vi "core_binary_split_DBL.vi"(9 "vector in":dbl[](array[numeric])) -> (0 "back":dbl[](array[numeric]), 1 "middle":dbl, 2 "front":dbl[](array[numeric]), 4 "odd length?":bool)   [LabVIEW 2015]
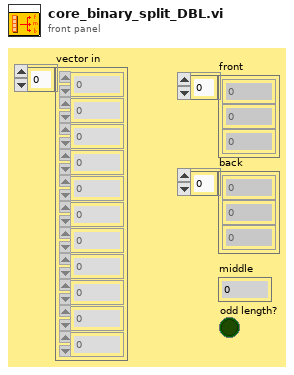
[diagram p1: front panel]
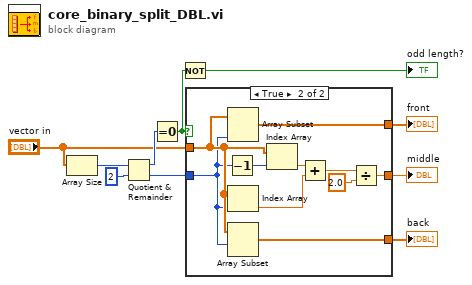
[diagram p0: block diagram]
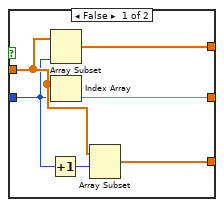
[diagram p2: hidden frame]
diagram:
  n1 = Array Size(array="vector in") -> (size(s)=w9:i32)
  n2 = Quotient & Remainder(x=w9, y=2) -> (x-y*floor(x/y)=w8:i32, floor(x/y)=w7:i32)
  n3 = Equal To 0?(x=w8) -> (x = 0?=w2:bool)
  n4 = Not(x=w2) -> (.not. x?=→"odd length?":bool)
  n5 = case shown="True" w2 {
    tunnel: "vector in" -> [w15 w24]
    tunnel: w7 -> [w14 w23]
    tunnel: [w13 w26] -> w5
    tunnel: [w12 w25] -> w4
    tunnel: [w11 w17] -> w3
    frame False {
      n6 = Increment(x=w14) -> (x+1=w16:i32)
      n7 = Array Subset(array=w15, length=w14) -> (w13:dbl[])  [unwired: 1 in]
      n8 = Index Array(array=w15, index=w14) -> (element=w11:dbl)
      n9 = Array Subset(array=w15, index=w16) -> (w12:dbl[])  [unwired: 1 in]
    }
    frame True {
      n10 = Decrement(x=w23) -> (x-1=w22:i32)
      n11 = Array Subset(array=w24, length=w23) -> (w26:dbl[])  [unwired: 1 in]
      n12 = Index Array(array=w24, index=w23) -> (element=w20:dbl)
      n13 = Array Subset(array=w24, index=w23) -> (w25:dbl[])  [unwired: 1 in]
      n14 = Index Array(array=w24, index=w22) -> (element=w21:dbl)
      n15 = Add(x=w21, y=w20) -> (x+y=w19:dbl)
      n16 = Divide(x=w19, y=2.0) -> (x/y=w17:dbl)
    }
  }
  "front" <- w5
  "back" <- w4
  "middle" <- w3
